vi "Main.vi"(11 "Module Admin":refnum<class "Delacor_lib_QMH_Module Admin.lvclass">) -> ()   [LabVIEW 2020, in "Config.lvlib"]
doc: "This template is based off of the Queued Message Handler design pattern and the Queued Message Handler project template that ships with LabVIEW.\n\nThe main difference is that the queue is private to this module and communication between modules is performed via Broadcast and Request events.\n\nRequest events are wrapped in public API methods and are handled in the Event Handling Loop (EHL) of this VI. Any module can register for Broadcast events sent by this module. The EHL generates messages based on user interface actions.\n\nThe Message Handling Loop (MHL) processes messages generated by the EHL, or by other messages. The messages are string values, so new messages can be added easily to the Message Cases case structure in the MHL. Each message cluster can also provide an optional value for Message Data, which is a variant that can be converted to whatever message-specific data is required.\n_____\nBased on Delacor QMH Project Template 5.0.0.82."
uses:
  Config.lvlib
  <vilib>/Delacor/Delacor QMH/Libraries/Module Admin_class/Delacor_lib_QMH_Module Admin.lvclass
  Module Data--cluster.ctl
  <vilib>/Delacor/Delacor QMH/Libraries/Message Queue_class/Delacor_lib_QMH_Message Queue.lvclass/Delacor_lib_QMH_Message Queue.ctl
  Stop Argument--cluster.ctl
  <vilib>/Utility/miscctls.llb/LVPointTypeDef.ctl
  <vilib>/Delacor/Delacor QMH/Libraries/Module Admin_class/Delacor_lib_QMH_Module Admin.lvclass/Delacor_lib_QMH_Module Admin.ctl
  <vilib>/Delacor/Delacor QMH/Libraries/Message Queue_class/Delacor_lib_QMH_Enqueue Message (Single).vi
  <vilib>/Delacor/Delacor QMH/Libraries/Module Admin_class/Delacor_lib_QMH_Get External Launch.vi
  <vilib>/Utility/error.llb/Error Cluster From Error Code.vi
  <vilib>/ErrorRing/Error Ring.xnode
  <vilib>/Delacor/Delacor QMH/Libraries/Message Queue_class/Delacor_lib_QMH_Message Queue.lvclass
  Acquisition whit helper loop/Acquisition whit helper loop.lvlib
  Logging/Logging.lvlib
panel:
  in  "Data":string
  in  "Config":T1={"frequency"=10.0, "square wave duty cycle (%)"=50.0, "phase"=0.0, "amplitude"=1.0, "signal type"=enum."Sine Wave", "offset"=0.0, "sampling info"={"Fs"=1000.0, "#s"=1000.0}}
  in  "Simulate MHL Error":bool
  in  "Simulate EHL Error":bool
  out "error out":errorcluster
  out "Status":string
  # "Config"
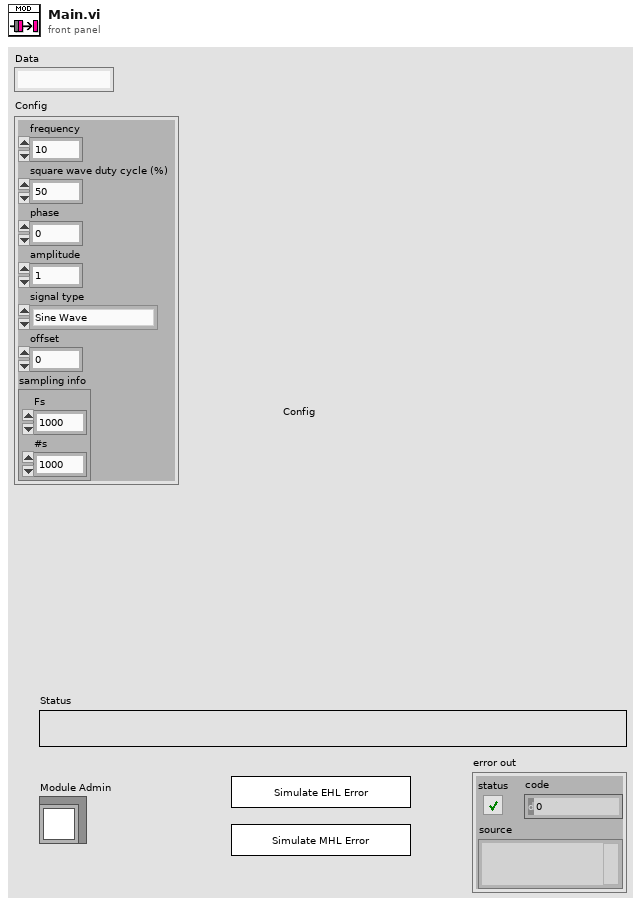
[diagram p1: front panel]
types:
  T1 = cluster{"frequency":dbl, "square wave duty cycle (%)":dbl, "phase":dbl, "amplitude":dbl, "signal type":enum16{"Sine Wave", "Triangle Wave", "Square Wave", "Sawtooth Wave"}, "offset":dbl, "sampling info":cluster{"Fs":dbl, "#s":dbl}}
  T2 = typedef "Config.lvlib/Request Events--cluster.ctl" = cluster{"Stop Module":refnum<user-event>, "Show Panel":refnum<user-event>, "Hide Panel":refnum<user-event>, "Get Module Execution Status":refnum<user-event>, "Show Diagram":refnum<user-event>}
  T3 = typedef "Config.lvlib/Module Data--cluster.ctl" = cluster{"Status":string}
  T4 = enum32{"invalid lock state", "Not Locked", "Locked (No Password)", "Password-protected"}
  T5 = typedef "Config.lvlib/Stop Argument--cluster.ctl" = cluster{"Origin":string, "Exit via Stop Module Req?":bool, "Wait for Module to stop?":bool}
  T6 = typedef "LVPointTypeDef.ctl" = cluster{"Horizontal":i16, "Vertical":i16}
  T7 = enum32{"Invalid", "Standard", "Closed", "Hidden", "Minimized", "Maximized"}
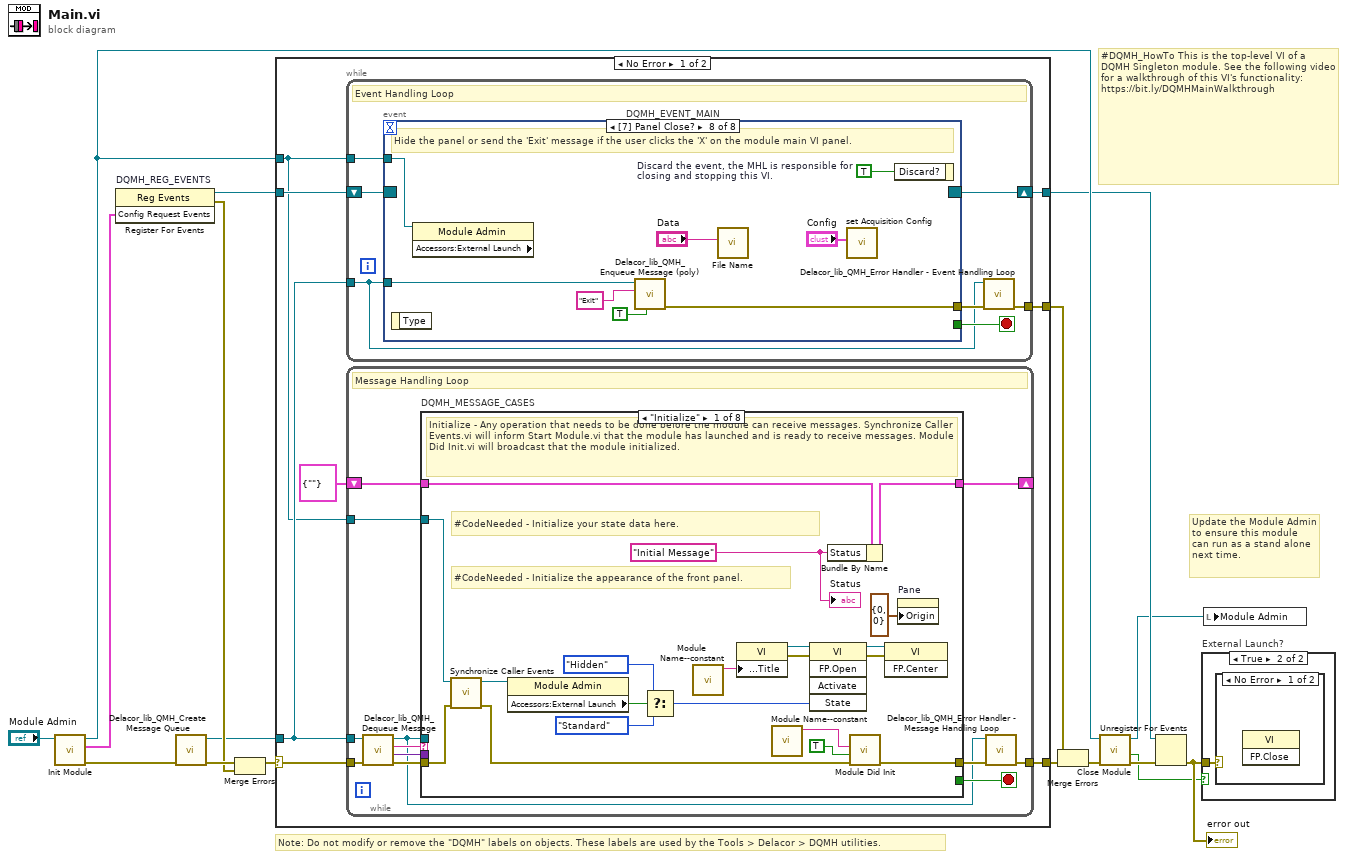
[diagram p0: block diagram]
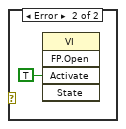
[diagram p3: hidden frame]
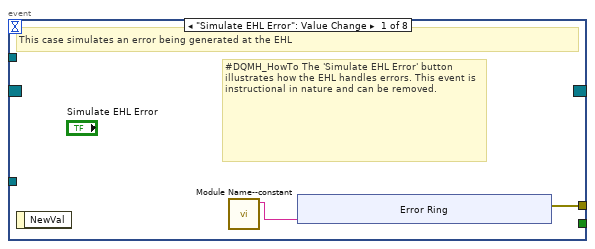
[diagram p4: hidden frame]
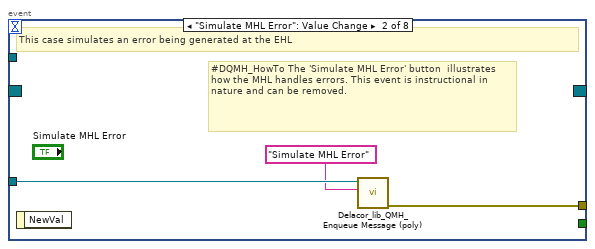
[diagram p5: hidden frame]
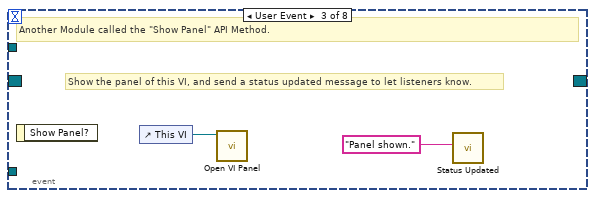
[diagram p6: hidden frame]
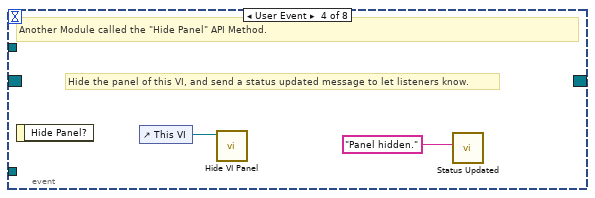
[diagram p7: hidden frame]
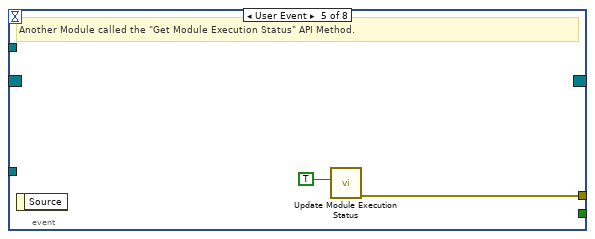
[diagram p8: hidden frame]
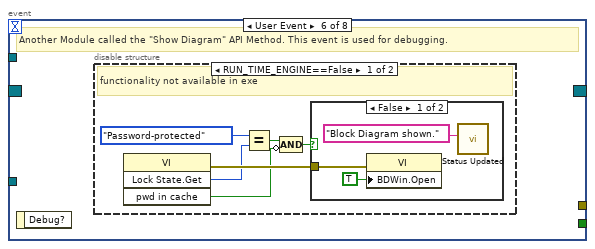
[diagram p9: hidden frame]
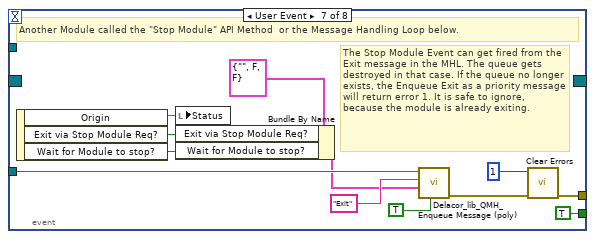
[diagram p12: hidden frame]
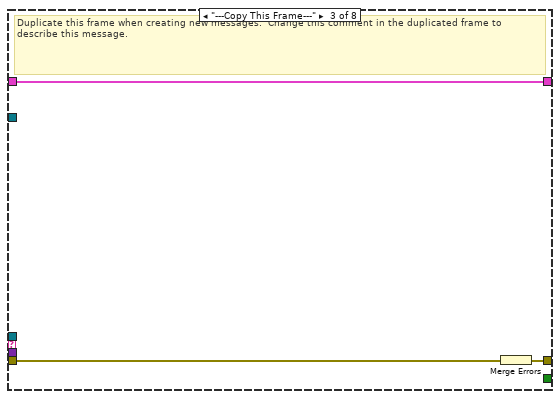
[diagram p14: hidden frame]
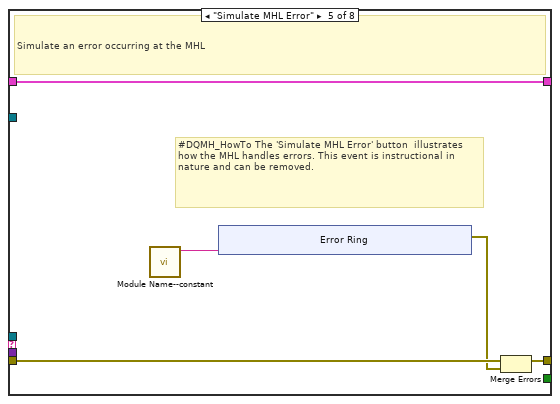
[diagram p16: hidden frame]
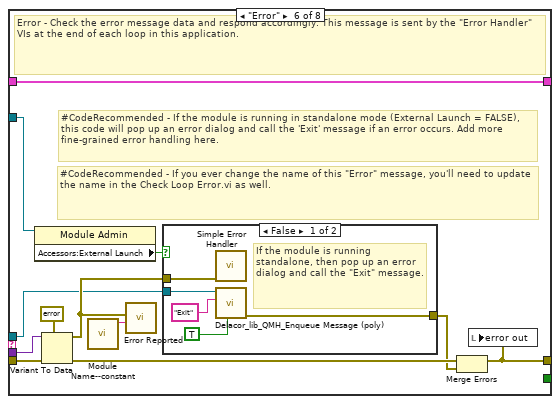
[diagram p17: hidden frame]
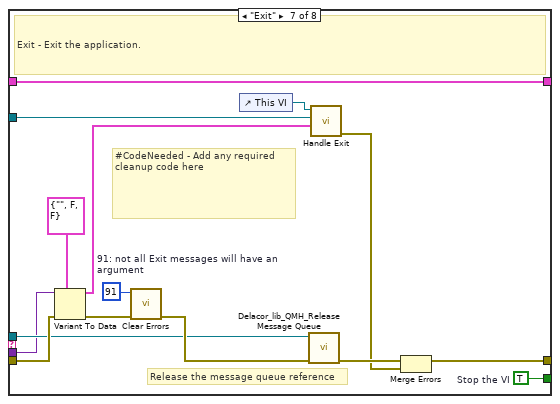
[diagram p19: hidden frame]
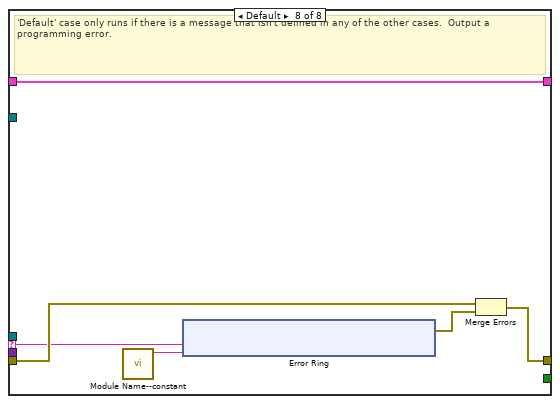
[diagram p20: hidden frame]
diagram:
  # "#DQMH_HowTo This is the top-level VI of a DQMH Singleton module. See the following video for a walkthrough of this VI's functionality: https://bit.ly/DQMHMainWalkthrough"
  # "Note: Do not modify or remove the \"DQMH\" labels on objects. These labels are used by the Tools > Delacor > DQMH utilities."
  # "Update the Module Admin to ensure this module can run as a stand alone next time."
  n1 = call "Init Module.vi"("Singleton Module Admin in"="Module Admin") -> ("error out"=w16:errorcluster, "Config Request Events"=w5:T2, "Singleton Module Admin out"=w8:refnum<class "Delacor_lib_QMH_Module Admin.lvclass">)  [unwired: 8 in]
  n2 = register-events "DQMH_REG_EVENTS"(w5) -> (reference out=w6:refnum<event-registration>, error out=w9:errorcluster)  [unwired: 2 in]
  n3 = call <vilib>:"Delacor_lib_QMH_Create Message Queue.vi"("error in (no error)"=w16) -> ("error out"=w11:errorcluster, "Message Queue"=w4:refnum<class "Delacor_lib_QMH_Message Queue.lvclass">)  [unwired: 9 in]
  n4 = Merge Errors(w11, w9) -> (w10:errorcluster)
  n5 = case shown="No Error" w10 {
    selector: w10 -> [w23 w179]
    tunnel: [w25 w178] -> w17
    tunnel: [w22 w184] -> w7
    tunnel: w6 -> [w20 w184]
    tunnel: w4 -> [w19 w177]
    tunnel: [w24 _] -> w14
    tunnel: w8 -> [w18 w180]
    frame No Error {
      n6 = while {
        tunnel: w19 -> [w26]
        shift-right: [w29] -> w22
        shift-left: w20 -> [w30]
        tunnel: [w31] -> w24
        tunnel: w18 -> [w27]
        stop <- w28 stop-if-true
        # "Event Handling Loop"
        n7 = event "DQMH_EVENT_MAIN" shown="[7] Panel Close?" {
          selector: w30 -> [_ _ _ _ _ _ _ _]
          dyn-events: [_ _ _ _ _ _ _ _] -> w29
          timeout: _ -> [_ _ _ _ _ _ _ _]
          tunnel: [_ _ _ _ _ _ TRUE ("Discard?") _] -> w28
          tunnel: w26 -> [_ w43 _ _ _ _ w67 w78]
          tunnel: [w34 w44 _ _ w50 _ w70 w72] -> w32
          tunnel: w27 -> [_ _ _ _ _ _ _ w77]
          event "Simulate EHL Error": Value Change {
            # "#DQMH_HowTo The 'Simulate EHL Error' button  illustrates how the EHL handles errors. This event is instructional in nature and can be removed."
            # "This case simulates an error being generated at the EHL"
            n8 = event-data() -> ()  [unwired: 1 in, 1 out]
            n9 = call "Module Name--constant.vi"() -> ("Module Name"=w33:string)  [unwired: 11 in]
            n10 = xnode "Error Ring"("parameter 0"=w33) -> ("error out"=w34:errorcluster)
          }
          event "Simulate MHL Error": Value Change {
            # "#DQMH_HowTo The 'Simulate MHL Error' button  illustrates how the MHL handles errors. This event is instructional in nature and can be removed."
            # "This case simulates an error being generated at the EHL"
            n11 = event-data() -> ()  [unwired: 1 in, 1 out]
            n12 = call-poly <vilib>:"Delacor_lib_QMH_Enqueue Message (poly).vi"("Message"="Simulate MHL Error", "Message Queue in"=w43) -> ("error out"=w44:errorcluster)  [unwired: 8 in, 1 out]
          }
          event User Event {
            # "Show the panel of this VI, and send a status updated message to let listeners know."
            # "Another Module called the \"Show Panel\" API Method."
            n13 = event-data() -> ()  [unwired: 1 in, 1 out]
            n14 = control-ref of="This VI"() -> (w46:refnum<vi>)
            n15 = call "Open VI Panel.vi"("VI"=w46) -> ()  [unwired: 10 in, 1 out]
            n16 = call "Status Updated.vi"("Status"="Panel shown." ("format string")) -> ()  [unwired: 10 in, 1 out]
          }
          event User Event {
            # "Hide the panel of this VI, and send a status updated message to let listeners know."
            # "Another Module called the \"Hide Panel\" API Method."
            n17 = event-data() -> ()  [unwired: 1 in, 1 out]
            n18 = control-ref of="This VI"() -> (w48:refnum<vi>)
            n19 = call "Hide VI Panel.vi"("VI"=w48) -> ()  [unwired: 10 in, 1 out]
            n20 = call "Status Updated.vi"("Status"="Panel hidden." ("format string")) -> ()  [unwired: 10 in, 1 out]
          }
          event User Event {
            # "Another Module called the \"Get Module Execution Status\" API Method."
            n21 = event-data() -> ()  [unwired: 1 in, 1 out]
            n22 = call "Update Module Execution Status.vi"("Running?"=TRUE) -> ("error out"=w50:errorcluster)  [unwired: 10 in]
          }
          event User Event {
            # "Another Module called the \"Show Diagram\" API Method. This event is used for debugging."
            n23 = event-data() -> ()  [unwired: 1 in, 1 out]
            n24 = disable-structure shown="RUN_TIME_ENGINE==False" {
              frame condition #0 (active) {
                # "functionality not available in exe"
                n25 = invoke class="VI" method="Lock State.Get"() -> (error out=w56:errorcluster, "Get Lock State"=w55:T4, "pwd in cache"=w52:bool)  [unwired: 4 in, 1 out]
                n26 = Equal?(x=T4."Password-protected", y=w55) -> (x = y?=w53:bool)
                n27 = Compound Arithmetic op=AND(w53, invert w52) -> (w51:bool)
                n28 = case shown="False" w51 {
                  tunnel: w56 -> [w59 _]
                  frame False {
                    n29 = property class="VI"(error in=w59, "BDWin.Open"=TRUE ("Block Diagram Window:Open")) -> ()  [unwired: 1 in, 2 out]
                    n30 = call "Status Updated.vi"("Status"="Block Diagram shown." ("format string")) -> ()  [unwired: 10 in, 1 out]
                  }
                  frame True {
                    # "Password-protected VI, and the password is not in the cache. Do not show the diagram."
                  }
                }
              }
              frame condition #1 {
              }
            }
          }
          event User Event {
            # "The Stop Module Event can get fired from the Exit message in the MHL. The queue gets destroyed in that case. If the queue no longer exists, the Enqueue Exit as a priority message will return error 1. It is safe to ignore, because the module is already exiting."
            # "Another Module called the \"Stop Module\" API Method  or the Message Handling Loop below."
            n31 = event-data() -> ("Origin"=w66:string, "Exit via Stop Module Req?"=w62:bool, "Wait for Module to stop?"=w61:bool)  [unwired: 1 in]
            n32 = local write "Status"(w66) -> ()
            n33 = Bundle By Name(cluster=T5 {"Origin"="", "Exit via Stop Module Req?"=FALSE, "Wait for Module to stop?"=FALSE} ("Stop Argument"), "Exit via Stop Module Req?"=w62, "Wait for Module to stop?"=w61) -> (w60:T5)
            n34 = call-poly <vilib>:"Delacor_lib_QMH_Enqueue Message (poly).vi"("Priority Message? (F)"=TRUE, "Message Data"=w60, "Message"="Exit", "Message Queue in"=w67) -> ("error out"=w71:errorcluster)  [unwired: 6 in, 1 out]
            n35 = call <vilib>:"Clear Errors.vi"("error in (no error)"=w71, "specific error code to clear (0: all)"=1) -> ("error out"=w70:errorcluster)  [unwired: 4 in, 1 out]
          }
          event Panel Close? {
            w79 = TRUE  # Discard the event, the MHL is responsible for closing and stopping this VI.
            # "Hide the panel or send the 'Exit' message if the user clicks the 'X' on the module main VI panel."
            n36 = event-data() -> ()  [unwired: 1 in, 1 out]
            n37 = property class="Module Admin" props=["Accessors:External Launch"](reference=w77) -> ()  [unwired: 1 in, 3 out]
            n38 = call-poly <vilib>:"Delacor_lib_QMH_Enqueue Message (poly).vi"("Priority Message? (F)"=TRUE, "Message"="Exit", "Message Queue in"=w78) -> ("error out"=w72:errorcluster)  [unwired: 7 in, 1 out]
            n39 = call "File Name.vi"("String"="Data") -> ()  [unwired: 10 in, 1 out]
            n40 = call "set Acquisition Config.vi"("Config"="Config") -> ()  [unwired: 10 in, 1 out]
            n41 = event-data("Discard?"=w79) -> ()  [unwired: 1 in, 1 out]
          }
        }
        n42 = call-dynamic "Delacor_lib_QMH_Error Handler - Event Handling Loop.vi"("error in (no error)"=w32, "Message Queue in"=w26) -> ("dup error in"=w31:errorcluster)  [unwired: 8 in, 1 out]
      }
      n43 = while {
        tunnel: w19 -> [w82]
        shift-right: [w86] -> _
        shift-left: T3 {"Status"=""} ("Data Cluster") -> [w87]
        tunnel: w23 -> [w90]
        tunnel: [w88] -> w25
        tunnel: w18 -> [w80]
        stop <- w85 stop-if-true
        # "Message Handling Loop"
        n44 = call-dynamic "Delacor_lib_QMH_Dequeue Message.vi"("error in (no error)"=w90, "Message Queue in"=w82) -> ("error out"=w89:errorcluster, "Message Data"=w83:variant, "Message"=w84:string, "Message Queue out"=w81:refnum<class "Delacor_lib_QMH_Message Queue.lvclass">)  [unwired: 6 in]
        n45 = case "DQMH_MESSAGE_CASES" shown="\"Initialize\"" w84 {
          selector: w84 -> [_ _ _ _ _ _ _ w164]
          tunnel: w81 -> [_ _ _ _ _ w134 w156 _]
          tunnel: w89 -> [w109 w113 w116 w118 w123 w141 w162 w166]
          tunnel: [w107 w113 w115 w118 w122 w137 w159 w167] -> w91
          tunnel: w87 -> [w98 w112 w114 w117 w120 w136 w155 w165]
          tunnel: [w97 w112 w114 w117 w120 w136 w155 w165] -> w86
          tunnel: [_ _ _ _ _ _ w154 _] -> w85
          tunnel: w83 -> [_ _ _ _ _ w135 w153 _]
          tunnel: w80 -> [w99 _ _ _ _ w133 w148 _]
          frame "Initialize" {
            w92 = "Initial Message" ("Initial Message")
            # "#CodeNeeded - Initialize the appearance of the front panel."
            # "#CodeNeeded - Initialize your state data here."
            # "Initialize - Any operation that needs to be done before the module can receive messages. Synchronize Caller Events.vi will inform Start Module.vi that the module has launched and is ready to receive messages. Module Did Init.vi will broadcast that the module initialized."
            n46 = call "Synchronize Caller Events.vi"("error in (no error)"=w109, "Singleton Module Admin in"=w99) -> ("error out"=w108:errorcluster, "Singleton Module Admin out"=w94:refnum<class "Delacor_lib_QMH_Module Admin.lvclass">)  [unwired: 8 in]
            n47 = property class="Module Admin"(reference=w94) -> ("Accessors:External Launch"=w103:bool)  [unwired: 1 in, 2 out]
            n48 = Select(t=T7."Hidden" ("State"), s=w103, f=T7."Standard" ("State")) -> (s? t:f=w100:T7)
            n49 = call "Module Name--constant.vi"() -> ("Module Name"=w106:string)  [unwired: 11 in]
            n50 = property class="VI"("Front Panel.Title"=w106) -> (reference out=w105:refnum<vi>, error out=w111:errorcluster)  [unwired: 2 in]
            n51 = call "Module Name--constant.vi"() -> ("Module Name"=w95:string)  [unwired: 11 in]
            n52 = invoke class="VI" method="FP.Open"(reference=w105, error in=w111, "State"=w100) -> (reference out=w104:refnum<vi>, error out=w110:errorcluster)  [unwired: 2 in, 3 out]
            n53 = Bundle By Name(cluster=w98, "Status"=w92) -> (w97:T3)
            n54 = call "Module Did Init.vi"("error in (no error)"=w108, "Initialized?"=TRUE, "Origin"=w95) -> ("error out"=w107:errorcluster)  [unwired: 8 in]
            n55 = invoke class="VI" method="FP.Center"(reference=w104, error in=w110) -> ()  [unwired: 1 in, 3 out]
            n56 = property on="Pane" class="Pane"("Origin"=T6 {"Horizontal"=0, "Vertical"=0}) -> ()  [unwired: 2 in, 2 out]
            "Status" <- w92
          }
          frame "--- Module Specific ---" {
            # "Separator -- The following cases handle messages specific to this Module."
          }
          frame "---Copy This Frame---" {
            # "Duplicate this frame when creating new messages.  Change this comment in the duplicated frame to describe this message."
            n57 = Merge Errors(w116) -> (w115:errorcluster)
          }
          frame "--- Exit and Error Handling---" {
            # "Separator - The following cases handle errors and exit messages."
          }
          frame "Simulate MHL Error" {
            # "#DQMH_HowTo The 'Simulate MHL Error' button  illustrates how the MHL handles errors. This event is instructional in nature and can be removed."
            # "Simulate an error occurring at the MHL"
            n58 = call "Module Name--constant.vi"() -> ("Module Name"=w119:string)  [unwired: 11 in]
            n59 = xnode "Error Ring"("parameter 0"=w119) -> ("error out"=w121:errorcluster)
            n60 = Merge Errors(w123, w121) -> (w122:errorcluster)
          }
          frame "Error" {
            # "#CodeRecommended - If you ever change the name of this \"Error\" message, you'll need to update the name in the Check Loop Error.vi as well."
            # "#CodeRecommended - If the module is running in standalone mode (External Launch = FALSE), this code will pop up an error dialog and call the 'Exit' message if an error occurs. Add more fine-grained error handling here."
            # "Error - Check the error message data and respond accordingly. This message is sent by the \"Error Handler\" VIs at the end of each loop in this application."
            n61 = property class="Module Admin"(reference=w133) -> ("Accessors:External Launch"=w132:bool)  [unwired: 1 in, 2 out]
            n62 = Variant To Data(error in=w141, type=errorcluster {"status"=FALSE, "code"=0, "source"=""} ("error constant"), Variant=w135) -> (data=w142:errorcluster, error out=w139:errorcluster)
            n63 = call "Module Name--constant.vi"() -> ("Module Name"=w131:string)  [unwired: 11 in]
            n64 = call "Error Reported.vi"("Additional Information"=w131, "Error"=w142) -> ()  [unwired: 9 in, 1 out]
            n65 = case shown="False" w132 {
              tunnel: [w147 _] -> w138
              tunnel: w134 -> [w145 _]
              tunnel: w142 -> [w146 _]
              frame False {
                # "If the module is running standalone, then pop up an error dialog and call the \"Exit\" message."
                n66 = call <vilib>:"Simple Error Handler.vi"("error in (no error)"=w146) -> ()  [unwired: 4 in, 5 out]
                n67 = call-poly <vilib>:"Delacor_lib_QMH_Enqueue Message (poly).vi"("Priority Message? (F)"=TRUE, "Message"="Exit", "Message Queue in"=w145) -> ("error out"=w147:errorcluster)  [unwired: 7 in, 1 out]
              }
              frame True {
                # "If the module was launched externally, calling the Error Reported broadcast VI is the only action performed by the \"Error\" message. The module's caller can then process the error appropriately."
              }
            }
            n68 = Merge Errors(w139, w138) -> (w137:errorcluster)
            n69 = local write "error out"(w137) -> ()
          }
          frame "Exit" {
            w152 = 91  # 91: not all Exit messages will have an argument
            w154 = TRUE  # Stop the VI
            # "Release the message queue reference"
            # "#CodeNeeded - Add any required cleanup code here"
            # "Exit - Exit the application."
            n70 = Variant To Data(error in=w162, type=T5 {"Origin"="", "Exit via Stop Module Req?"=FALSE, "Wait for Module to stop?"=FALSE} ("Stop Argument"), Variant=w153) -> (data=w150:T5, error out=w158:errorcluster)
            n71 = call <vilib>:"Clear Errors.vi"("error in (no error)"=w158, "specific error code to clear (0: all)"=w152) -> ("error out"=w161:errorcluster)  [unwired: 4 in, 1 out]
            n72 = control-ref of="This VI"() -> (w149:refnum<vi>)
            n73 = call-dynamic "Delacor_lib_QMH_Release Message Queue.vi"("error in (no error)"=w161, "Message Queue"=w156) -> ("error out"=w160:errorcluster)  [unwired: 9 in]
            n74 = call "Handle Exit.vi"("Stop Argument"=w150, "Admin in"=w148, "VI reference"=w149) -> ("error out"=w157:errorcluster)  [unwired: 7 in, 1 out]
            n75 = Merge Errors(w160, w157) -> (w159:errorcluster)
          }
          frame Default {
            # "'Default' case only runs if there is a message that isn't defined in any of the other cases.  Output a programming error."
            n76 = call "Module Name--constant.vi"() -> ("Module Name"=w163:string)  [unwired: 11 in]
            n77 = xnode "Error Ring"("parameter 0"=w164, "parameter 1"=w163) -> ("error out"=w168:errorcluster)
            n78 = Merge Errors(w166, w168) -> (w167:errorcluster)
          }
        }
        n79 = call-dynamic "Delacor_lib_QMH_Error Handler - Message Handling Loop.vi"("error in (no error)"=w91, "Message Queue in"=w81) -> ("dup error in"=w88:errorcluster)  [unwired: 8 in, 1 out]
      }
    }
    frame Error {
      # "Synchronize Caller Events.vi will inform Start Module.vi that the module has launched and will let the code calling Start Module.vi register for broadcasts and would permit the caller receive the broadcast that an error occurred at launch time."
      n80 = call-dynamic "Delacor_lib_QMH_Release Message Queue.vi"("error in (no error)"=w179, "Message Queue"=w177) -> ("error out"=w178:errorcluster)  [unwired: 9 in]
      n81 = call "Synchronize Caller Events.vi"("Singleton Module Admin in"=w180) -> ("error out"=w185:errorcluster)  [unwired: 9 in, 1 out]
      n82 = call "Module Name--constant.vi"() -> ("Module Name"=w183:string)  [unwired: 11 in]
      n83 = Format Into String(format string="An error occurred during initialization. %s is no longer running.", w183) -> (resulting string=w181:string)  [unwired: 2 in, 1 out]
      n84 = Merge Errors(w178, w185) -> (w186:errorcluster)
      n85 = call "Error Reported.vi"("Additional Information"=w181, "Error"=w186) -> ()  [unwired: 9 in, 1 out]
    }
  }
  n86 = Merge Errors(w14, w17) -> (w13:errorcluster)
  n87 = call "Close Module.vi"("error in (no error)"=w13, "Module Admin in"=w8) -> ("error out"=w15:errorcluster, "External Launch"=w1:bool, "Module Admin out"=w2:refnum<class "Delacor_lib_QMH_Module Admin.lvclass">)  [unwired: 7 in]
  n88 = Unregister For Events(event registration refnum=w7, error in=w15) -> (error out=w12:errorcluster)
  "error out" <- w12
  n89 = case "External Launch?" shown="True" w1 {
    tunnel: w12 -> [_ w187]
    frame False {
    }
    frame True {
      n90 = case shown="No Error" w187 {
        frame No Error {
          n91 = invoke class="VI" method="FP.Close"() -> ()  [unwired: 3 in, 3 out]
        }
        frame Error {
          n92 = invoke class="VI" method="FP.Open"("Activate"=TRUE ("Activate?")) -> ()  [unwired: 4 in, 5 out]
        }
      }
    }
  }
  n93 = local write "Module Admin"(w2) -> ()
